vi "Initialize.vi"(7 "ChannelName":string="Setpoint.ch%d.SP", 8 "error in":errorcluster, 9 "Number of Channels":u32=1, 10 "Instance Name":string, 11 "Parallel Mode Channels in":refnum<class "Parallel Mode Channels.lvclass">) -> (0 "error out":errorcluster, 3 "Parallel Mode Channels out":refnum<class "Parallel Mode Channels.lvclass">)   [LabVIEW 2023, in "Parallel Mode Channels.lvclass"]
uses:
  Parallel Mode Channels.lvclass
  Parallel Mode Channels.lvclass/Parallel Mode Channels.ctl
  <vilib>/ADAS Replay HIL/Channels/Tag Wrapper/Polymorphic/Open Consumer Tag (U16).vi
  <vilib>/ADAS Replay HIL/Channels/Tag Wrapper/Polymorphic/Set Default Value (U16).vi
  <vilib>/ADAS Replay HIL/Channels/Tag Wrapper/Polymorphic/Open Producer Tag (I32).vi
  <vilib>/ADAS Replay HIL/Channels/Tag Wrapper/Polymorphic/Set Default Value (I32).vi
  <vilib>/ADAS Replay HIL/Channels/Tag Wrapper/Polymorphic/Open Consumer Tag (Boolean).vi
  <vilib>/ADAS Replay HIL/Channels/Tag Wrapper/Polymorphic/Set Default Value (Boolean).vi
  <vilib>/ADAS Replay HIL/Channels/Tag Wrapper/Polymorphic/Open Consumer Tag (U16).vi/bacb721e-673a-491a-accd-959f2e1f334e.vi
  <vilib>/ADAS Replay HIL/Channels/Tag Wrapper/Polymorphic/Set Default Value (U16).vi/228e99de-6fcf-414d-86fc-dc277c7b351f.vi
  <vilib>/ADAS Replay HIL/Channels/Tag Wrapper/Polymorphic/Open Producer Tag (I32).vi/45cd6eaa-a1ce-41a4-8aba-62a49d103d7e.vi
  <vilib>/ADAS Replay HIL/Channels/Tag Wrapper/Polymorphic/Set Default Value (I32).vi/228e99de-6fcf-414d-86fc-dc277c7b351f.vi
  <vilib>/ADAS Replay HIL/Channels/Tag Wrapper/Polymorphic/Open Consumer Tag (Boolean).vi/bacb721e-673a-491a-accd-959f2e1f334e.vi
  <vilib>/ADAS Replay HIL/Channels/Tag Wrapper/Polymorphic/Set Default Value (Boolean).vi/228e99de-6fcf-414d-86fc-dc277c7b351f.vi
  <vilib>/ADAS Replay HIL/Channels/Tag Wrapper/Polymorphic/Open Consumer Tag (U16).vi/bacb721e-673a-491a-accd-959f2e1f334e.vi/c28b0ead-42ad-4072-80a2-aca7f2bd7ce3.vi
  <vilib>/ADAS Replay HIL/Channels/Tag Wrapper/Polymorphic/Set Default Value (U16).vi/228e99de-6fcf-414d-86fc-dc277c7b351f.vi/4bc1c15b-36ab-481f-b8dd-c64075ce723a.vi
  <vilib>/ADAS Replay HIL/Channels/Tag Wrapper/Polymorphic/Open Producer Tag (I32).vi/45cd6eaa-a1ce-41a4-8aba-62a49d103d7e.vi/c28b0ead-42ad-4072-80a2-aca7f2bd7ce3.vi
  <vilib>/ADAS Replay HIL/Channels/Tag Wrapper/Polymorphic/Set Default Value (I32).vi/228e99de-6fcf-414d-86fc-dc277c7b351f.vi/4bc1c15b-36ab-481f-b8dd-c64075ce723a.vi
  <vilib>/ADAS Replay HIL/Channels/Tag Wrapper/Polymorphic/Open Consumer Tag (Boolean).vi/bacb721e-673a-491a-accd-959f2e1f334e.vi/c28b0ead-42ad-4072-80a2-aca7f2bd7ce3.vi
  <vilib>/ADAS Replay HIL/Channels/Tag Wrapper/Polymorphic/Set Default Value (Boolean).vi/228e99de-6fcf-414d-86fc-dc277c7b351f.vi/4bc1c15b-36ab-481f-b8dd-c64075ce723a.vi
  <vilib>/ADAS Replay HIL/AdasHilServices/AdasHilServices Fill In Error Info Ex.vi
  <vilib>/ADAS Replay HIL/Channels/Tag Wrapper/Tag Wrapper.lvlib
  Utilities/Utilities.lvlib
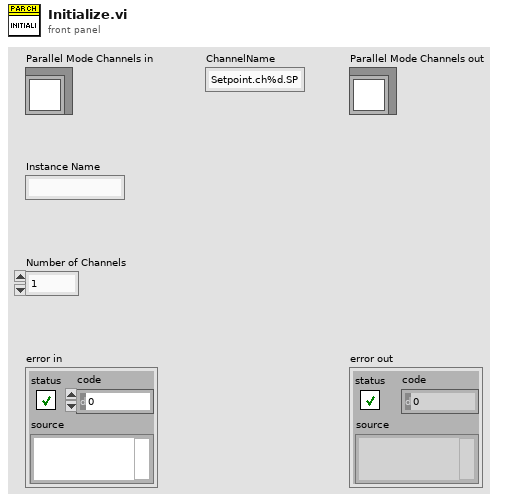
[diagram p1: front panel]
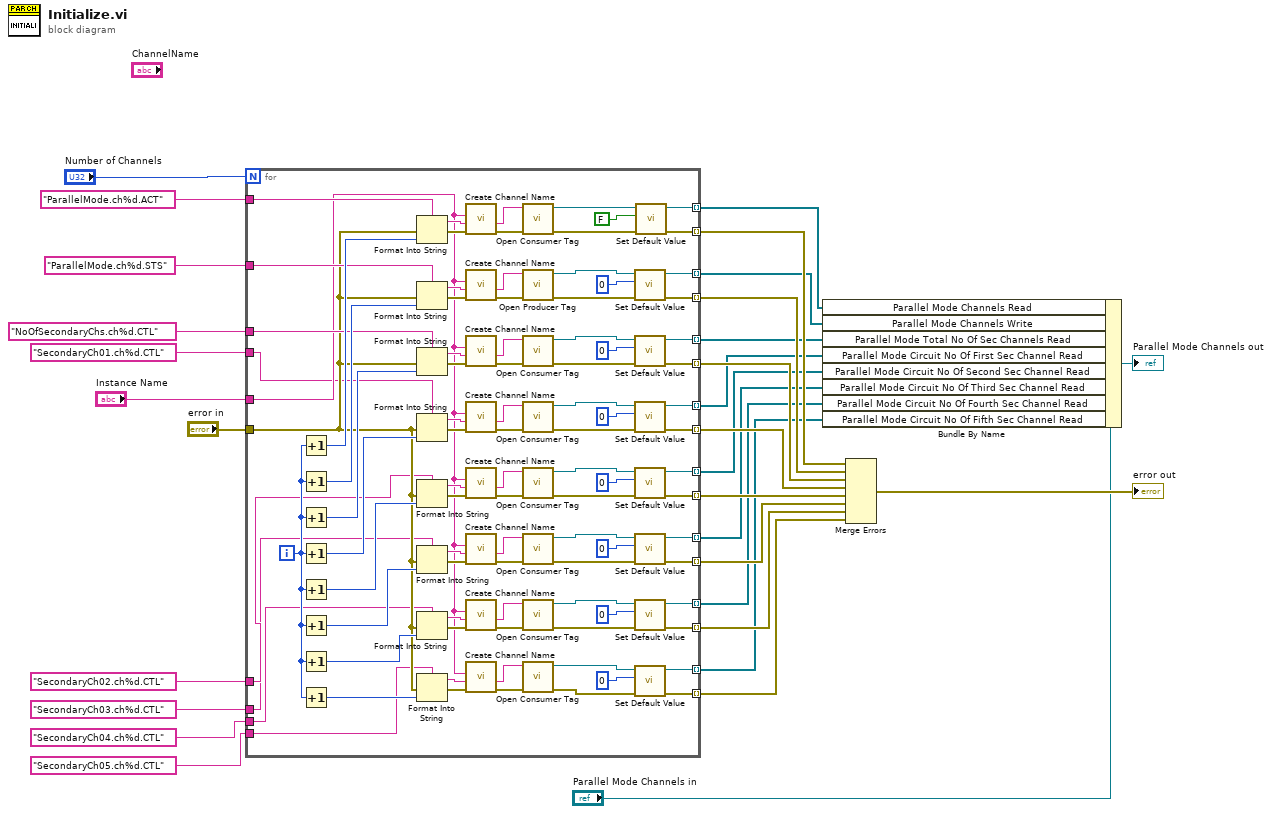
[diagram p0: block diagram]
diagram:
  n1 = for {
    N: "Number of Channels" -> [_]
    tunnel: "ParallelMode.ch%d.ACT" ("ChannelName") -> [w120]
    tunnel: "Instance Name" -> [w47]
    tunnel: "error in" -> [w48]
    tunnel: [w114] -> w29 mode=indexing
    tunnel: [w110] -> w28 mode=indexing
    tunnel: "ParallelMode.ch%d.STS" ("ChannelName") -> [w107]
    tunnel: [w105] -> w25 mode=indexing
    tunnel: [w104] -> w24 mode=indexing
    tunnel: "NoOfSecondaryChs.ch%d.CTL" ("ChannelName") -> [w91]
    tunnel: [w90] -> w17 mode=indexing
    tunnel: [w89] -> w16 mode=indexing
    tunnel: [w46] -> w15 mode=indexing
    tunnel: [w45] -> w14 mode=indexing
    tunnel: [w44] -> w13 mode=indexing
    tunnel: [w43] -> w12 mode=indexing
    tunnel: [w42] -> w11 mode=indexing
    tunnel: "SecondaryCh01.ch%d.CTL" ("ChannelName") -> [w40]
    tunnel: "SecondaryCh02.ch%d.CTL" ("ChannelName") -> [w39]
    tunnel: "SecondaryCh05.ch%d.CTL" ("ChannelName") -> [w38]
    tunnel: "SecondaryCh04.ch%d.CTL" ("ChannelName") -> [w37]
    tunnel: "SecondaryCh03.ch%d.CTL" ("ChannelName") -> [w36]
    tunnel: [w35] -> w5 mode=indexing
    tunnel: [w34] -> w4 mode=indexing
    tunnel: [w33] -> w3 mode=indexing
    tunnel: [w32] -> w2 mode=indexing
    tunnel: [w31] -> w1 mode=indexing
    i -> [w41]
    n2 = Increment(x=w41) -> (x+1=w121:i32)
    n3 = Increment(x=w41) -> (x+1=w108:i32)
    n4 = Increment(x=w41) -> (x+1=w99:i32)
    n5 = Increment(x=w41) -> (x+1=w88:i32)
    n6 = Increment(x=w41) -> (x+1=w80:i32)
    n7 = Increment(x=w41) -> (x+1=w72:i32)
    n8 = Increment(x=w41) -> (x+1=w64:i32)
    n9 = Increment(x=w41) -> (x+1=w56:i32)
    n10 = Format Into String(format string=w120, error in=w48, w121) -> (resulting string=w119:string, error out=w102:errorcluster)  [unwired: 1 in]
    n11 = Format Into String(format string=w107, error in=w48, w108) -> (resulting string=w106:string, error out=w101:errorcluster)  [unwired: 1 in]
    n12 = Format Into String(format string=w91, error in=w48, w99) -> (resulting string=w98:string, error out=w93:errorcluster)  [unwired: 1 in]
    n13 = Format Into String(format string=w40, error in=w48, w88) -> (resulting string=w87:string, error out=w82:errorcluster)  [unwired: 1 in]
    n14 = Format Into String(format string=w39, error in=w48, w80) -> (resulting string=w79:string, error out=w74:errorcluster)  [unwired: 1 in]
    n15 = Format Into String(format string=w36, error in=w48, w72) -> (resulting string=w71:string, error out=w66:errorcluster)  [unwired: 1 in]
    n16 = Format Into String(format string=w37, error in=w48, w64) -> (resulting string=w63:string, error out=w58:errorcluster)  [unwired: 1 in]
    n17 = Format Into String(format string=w38, error in=w48, w56) -> (resulting string=w55:string, error out=w50:errorcluster)  [unwired: 1 in]
    n18 = call "Create Channel Name.vi"("error in"=w102, "Channel Name"=w119, "Plugin Name"=w47) -> ("error out"=w103:errorcluster, "Data Channel Name"=w118:string)  [unwired: 7 in]
    n19 = call "Create Channel Name.vi"("error in"=w101, "Channel Name"=w106, "Plugin Name"=w47) -> ("error out"=w112:errorcluster, "Data Channel Name"=w109:string)  [unwired: 7 in]
    n20 = call "Create Channel Name.vi"("error in"=w93, "Channel Name"=w98, "Plugin Name"=w47) -> ("error out"=w94:errorcluster, "Data Channel Name"=w97:string)  [unwired: 7 in]
    n21 = call "Create Channel Name.vi"("error in"=w82, "Channel Name"=w87, "Plugin Name"=w47) -> ("error out"=w83:errorcluster, "Data Channel Name"=w86:string)  [unwired: 7 in]
    n22 = call "Create Channel Name.vi"("error in"=w74, "Channel Name"=w79, "Plugin Name"=w47) -> ("error out"=w75:errorcluster, "Data Channel Name"=w78:string)  [unwired: 7 in]
    n23 = call "Create Channel Name.vi"("error in"=w66, "Channel Name"=w71, "Plugin Name"=w47) -> ("error out"=w67:errorcluster, "Data Channel Name"=w70:string)  [unwired: 7 in]
    n24 = call "Create Channel Name.vi"("error in"=w58, "Channel Name"=w63, "Plugin Name"=w47) -> ("error out"=w59:errorcluster, "Data Channel Name"=w62:string)  [unwired: 7 in]
    n25 = call "Create Channel Name.vi"("error in"=w50, "Channel Name"=w55, "Plugin Name"=w47) -> ("error out"=w51:errorcluster, "Data Channel Name"=w54:string)  [unwired: 7 in]
    n26 = call-poly <vilib>:"Open Consumer Tag.vi"("error in"=w103, "Channel Name"=w118) -> ("error out"=w116:errorcluster, "ADAS HIL Channel"=w117:refnum<k21>)  [unwired: 8 in]
    n27 = call-poly <vilib>:"Open Producer Tag.vi"("error in"=w112, "Channel Name"=w109) -> ("error out"=w111:errorcluster, "ADAS HIL Channel"=w113:refnum<k21>)  [unwired: 8 in]
    n28 = call-poly <vilib>:"Open Consumer Tag.vi"("error in"=w94, "Channel Name"=w97) -> ("error out"=w95:errorcluster, "ADAS HIL Channel"=w96:refnum<k21>)  [unwired: 8 in]
    n29 = call-poly <vilib>:"Open Consumer Tag.vi"("error in"=w83, "Channel Name"=w86) -> ("error out"=w84:errorcluster, "ADAS HIL Channel"=w85:refnum<k21>)  [unwired: 8 in]
    n30 = call-poly <vilib>:"Open Consumer Tag.vi"("error in"=w75, "Channel Name"=w78) -> ("error out"=w76:errorcluster, "ADAS HIL Channel"=w77:refnum<k21>)  [unwired: 8 in]
    n31 = call-poly <vilib>:"Open Consumer Tag.vi"("error in"=w67, "Channel Name"=w70) -> ("error out"=w68:errorcluster, "ADAS HIL Channel"=w69:refnum<k21>)  [unwired: 8 in]
    n32 = call-poly <vilib>:"Open Consumer Tag.vi"("error in"=w59, "Channel Name"=w62) -> ("error out"=w60:errorcluster, "ADAS HIL Channel"=w61:refnum<k21>)  [unwired: 8 in]
    n33 = call-poly <vilib>:"Open Consumer Tag.vi"("error in"=w51, "Channel Name"=w54) -> ("error out"=w52:errorcluster, "ADAS HIL Channel"=w53:refnum<k21>)  [unwired: 8 in]
    n34 = call-poly <vilib>:"Set Default Value.vi"("error in"=w111, "Default Value"=0, "ADAS HIL Channel in"=w113) -> ("error out"=w110:errorcluster, "ADAS HIL Channel out"=w104:refnum<k21>)  [unwired: 7 in]
    n35 = call-poly <vilib>:"Set Default Value.vi"("error in"=w95, "Default Value"=u16 0, "ADAS HIL Channel in"=w96) -> ("error out"=w90:errorcluster, "ADAS HIL Channel out"=w89:refnum<k21>)  [unwired: 7 in]
    n36 = call-poly <vilib>:"Set Default Value.vi"("error in"=w84, "Default Value"=u16 0, "ADAS HIL Channel in"=w85) -> ("error out"=w46:errorcluster, "ADAS HIL Channel out"=w35:refnum<k21>)  [unwired: 7 in]
    n37 = call-poly <vilib>:"Set Default Value.vi"("error in"=w76, "Default Value"=u16 0, "ADAS HIL Channel in"=w77) -> ("error out"=w45:errorcluster, "ADAS HIL Channel out"=w34:refnum<k21>)  [unwired: 7 in]
    n38 = call-poly <vilib>:"Set Default Value.vi"("error in"=w68, "Default Value"=u16 0, "ADAS HIL Channel in"=w69) -> ("error out"=w44:errorcluster, "ADAS HIL Channel out"=w33:refnum<k21>)  [unwired: 7 in]
    n39 = call-poly <vilib>:"Set Default Value.vi"("error in"=w60, "Default Value"=u16 0, "ADAS HIL Channel in"=w61) -> ("error out"=w43:errorcluster, "ADAS HIL Channel out"=w32:refnum<k21>)  [unwired: 7 in]
    n40 = call-poly <vilib>:"Set Default Value.vi"("error in"=w52, "Default Value"=u16 0, "ADAS HIL Channel in"=w53) -> ("error out"=w42:errorcluster, "ADAS HIL Channel out"=w31:refnum<k21>)  [unwired: 7 in]
    n41 = call-poly <vilib>:"Set Default Value.vi"("error in"=w116, "Default Value"=FALSE, "ADAS HIL Channel in"=w117) -> ("error out"=w114:errorcluster, "ADAS HIL Channel out"=w105:refnum<k21>)  [unwired: 7 in]
  }
  n42 = Bundle By Name(cluster="Parallel Mode Channels in", "Parallel Mode Channels Read"=w25, "Parallel Mode Channels Write"=w24, "Parallel Mode Total No Of Sec Channels Read"=w16, "Parallel Mode Circuit No Of First Sec Channel Read"=w5, "Parallel Mode Circuit No Of Second Sec Channel Read"=w4, "Parallel Mode Circuit No Of Third Sec Channel Read"=w3, "Parallel Mode Circuit No Of Fourth Sec Channel Read"=w2, "Parallel Mode Circuit No Of Fifth Sec Channel Read"=w1) -> (→"Parallel Mode Channels out":refnum<class "Parallel Mode Channels.lvclass">)
  n43 = Merge Errors(w29, w28, w17, w15, w14, w13, w12, w11) -> (→"error out":errorcluster)
